vi "KickToSkill.vi"(0 "KickToSkill in":refnum<class "KickToSkill.lvclass">, 1 "use criteria?":bool, 2 "chipKick ?":bool, 5 "Robot":refnum<class "Robot.lvclass">, 9 "Game":refnum<class "Game.lvclass">, 10 "calculate force?":bool, 11 "error in (no error)":errorcluster, 12 "Target":dbl[](array[numeric]), 13 "KickForce 0?":bool) -> (4 "KickToSkill out":refnum<class "KickToSkill.lvclass">, 6 "Robot out":refnum<class "Robot.lvclass">, 15 "error out":errorcluster)   [LabVIEW 2020, in "KickToSkill.lvclass"]
uses:
  KickToSkill.lvclass
  Robot_class/Robot.lvclass
  Game_class/Game.lvclass
  Robot_class/roles.ctl
  Team_class/OffensivePlay.ctl
  Utilities_class/Utilities.lvclass
  Object_class/Object.lvclass/Object.ctl
  Robot_class/Robot.lvclass/Robot.ctl
  Game_class/Game.lvclass/Game.ctl
  Ball_class/Ball.lvclass/Ball.ctl
  Parameters_class/Parameters.lvclass/Parameters.ctl
  Team_class/Team.lvclass/Team.ctl
  <vilib>/Analysis/_algsub.llb/Real Vector Norm.vi
  <vilib>/Analysis/baseanly.llb/Real Dot Product.vi
  <vilib>/Analysis/coordinate.llb/2D Cartesian Coordinate Rotation (Scalar).vi
  Parameters_class/Read ChipKick Force 1.vi
  Team_class/Read OffensivePlay.vi
  Object_class/Read x.vi
  Robot_class/Write dest_x.vi
  Robot_class/Write dest_y.vi
  Robot_class/Write dest_orientation.vi
  Robot_class/Write kick_x.vi
  Robot_class/Write dest_x_kick.vi
  Robot_class/Write dest_y_kick.vi
  Robot_class/Write kick_z.vi
  Robot_class/Write dribble.vi
  Game_class/Read BallRef.vi
  Game_class/Read Parameters.lvclass.vi
  Game_class/Read FieldRef.vi
  Game_class/Read OffensiveTeam.vi
  Game_class/Read Utilities.lvclass.vi
  Game_class/Read EnemyRef.vi
  Parameters_class/Read ShootOutForce.vi
  Parameters_class/Read AttakingOurselves.vi
  Parameters_class/Read KickEps.vi
  Parameters_class/Read KickRange.vi
  Parameters_class/Read MinDistToKick.vi
  Parameters_class/Read DistanceToKickingAngle.vi
  Parameters_class/Read Force++.vi
  Parameters_class/Read ChipKick activated.vi
  Parameters_class/Read KickAngle.vi
  Parameters_class/Read DistanceToGoAroundBall.vi
  Parameters_class/Read KickForce.vi
  Parameters_class/Read Shoot Out_.vi
  Object_class/Read y.vi
  Ball_class/Read v_x.vi
  Ball_class/Read v_y.vi
  Robot_class/Read role.vi
  Robot_class/Read orientation.vi
  Ally_class/Ally.lvclass
  Ball_class/Ball.lvclass
  Parameters_class/Parameters.lvclass
  Field_class/Field.lvclass
  Enemy_class/Enemy.lvclass
  <vilib>/Analysis/NI_AALPro.lvlib
  <vilib>/Analysis/NI_AALBase.lvlib
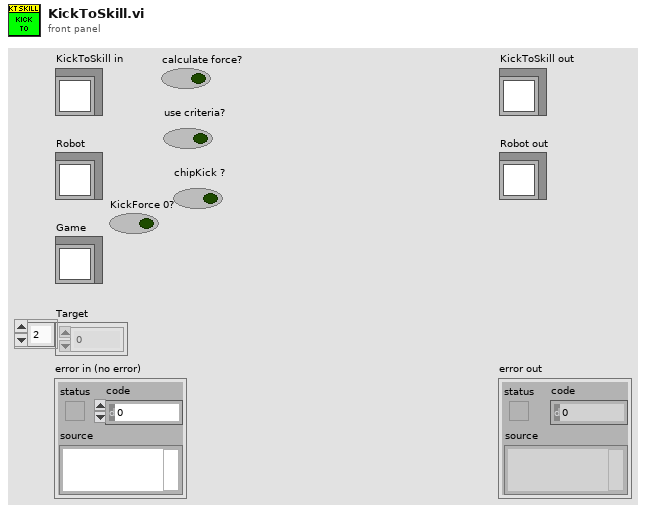
[diagram p1: front panel]
types:
  T1 = typedef "OffensivePlay.ctl" = enum16{"ABCPass", "PrepareTriplePass", "TableWithStriker", "TableWith2ndStrikerPlay", "PrepareDoublePass", "PrepareRollToPass", "SimplePass", "PreparePass", "PassToStriker", "BallOutOfField", "PassTo2ndStriker", "StopOffensive", "Prepare Penalty Enemy", "EnemyPossessionAtEnemyField", "EnemyPossesionAtOurField", "TestPlay", "PreparePenaltyAlly", "KickPenaltyAlly", "PrepareKickoffAlly", "PrepareKickoffEnemy", "IndirectEnemy", "DirectEnemy", "PreparePassInGame1", "NormalGame", "DirectKick", "Pass", "Halt", "Timeout", "PassPlay", "PenaltyEnemy"}
  T2 = typedef "roles.ctl" = enum16{"ABCThirdKicker", "ABCFirstKicker", "ABCSecondKicker", "Tabler", "TableFinalizer", "PrepareRollToPassRoller", "PrepareRollToPassReceiver", "SimplePassRoll", "SimplePassRollReceiver", "PenaltyDefense", "PreparePassReceiver 2", "PreparePassReceiver 1", "PassObserver", "Timeout", "Goto", "ZigZag", "None", "BallOutOfField", "DefenderArea", "Duelist", "AttackerStop", "FollowAttacker", "KeeperRole", "KickPenalty", "AttackerAimGoal", "AttackerBlock", "Marker", "Halt", "Shoot", "PassKicker", "PassReceiver", "TestRole", "PenaltyAttacker"}
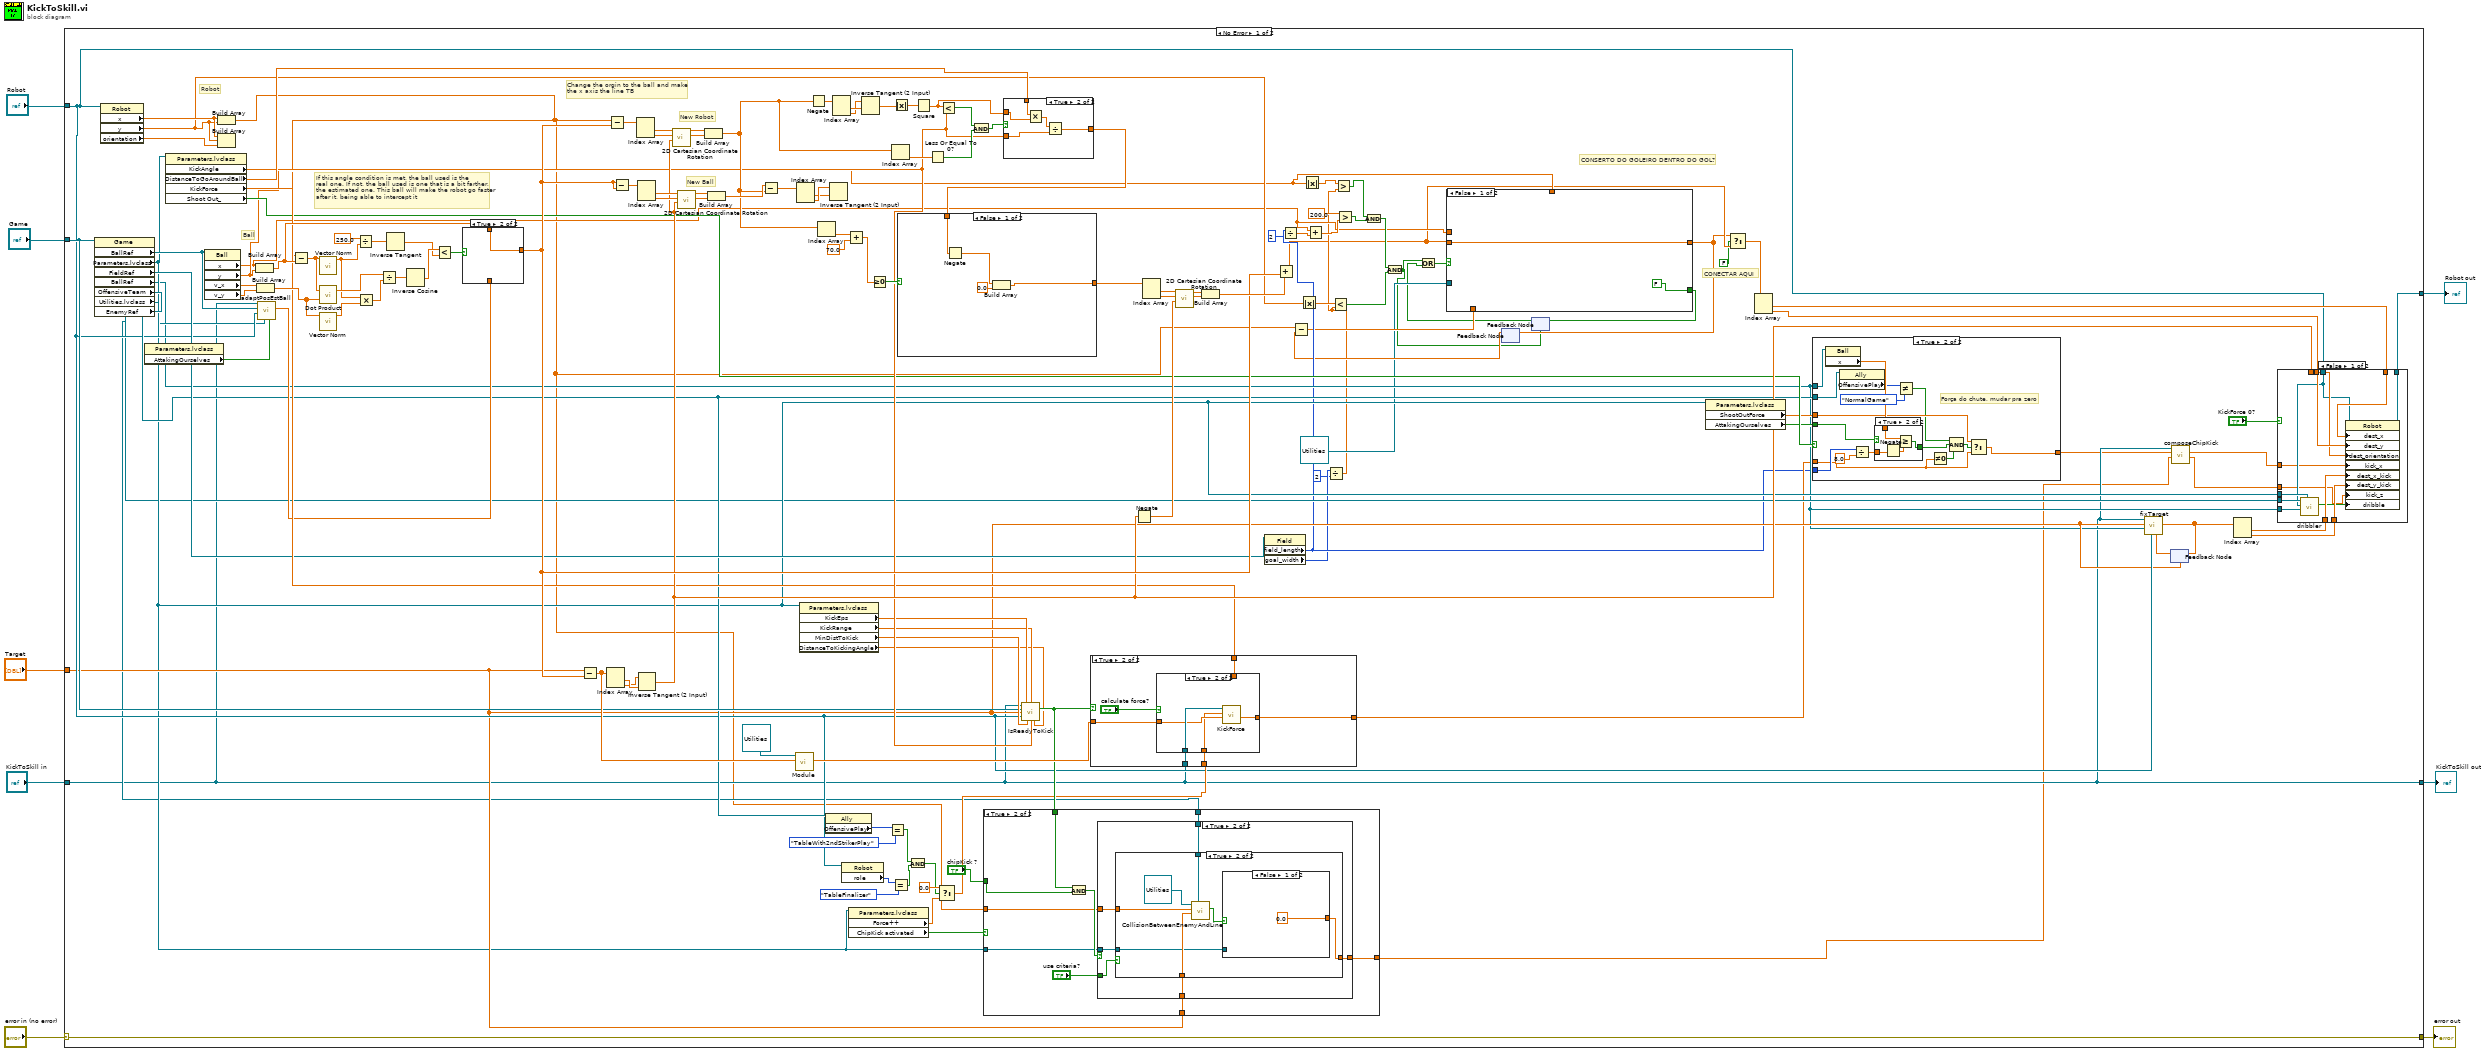
[diagram p0: block diagram]
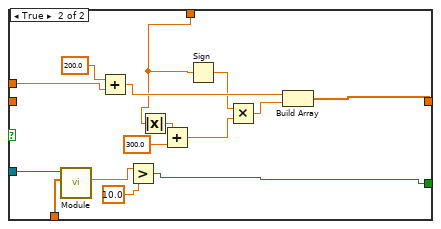
[diagram p2: hidden frame]
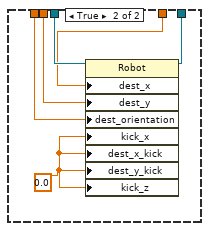
[diagram p3: hidden frame]
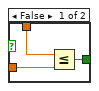
[diagram p5: hidden frame]
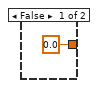
[diagram p6: hidden frame]
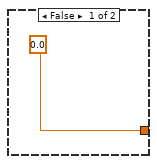
[diagram p7: hidden frame]
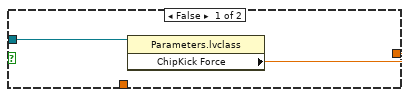
[diagram p8: hidden frame]
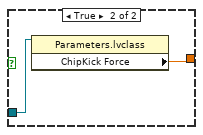
[diagram p9: hidden frame]
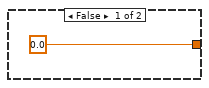
[diagram p10: hidden frame]
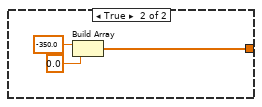
[diagram p12: hidden frame]
diagram:
  n1 = case shown="No Error" "error in (no error)" {
    selector: "error in (no error)" -> [w148 w267]
    tunnel: [w148 w267] -> w7
    tunnel: [w42 w266] -> w5
    tunnel: "KickToSkill in" -> [w42 w266]
    tunnel: "Robot" -> [w52 w265]
    tunnel: "Game" -> [w70 _]
    tunnel: "Target" -> [w49 _]
    tunnel: [w89 w265] -> w1
    frame No Error {
      # "CONECTAR AQUI"
      # "CONSERTO DO GOLEIRO DENTRO DO GOL?"
      # "Change the orgin to the ball and make \nthe x axis the line TB"
      # "If this angle condition is met, the ball used is the\nreal one. If not, the ball used is one that is a bit farther,\nthe estimated one. This ball will make the robot go faster\nafter it, being able to intercept it"
      # "New Robot"
      # "New Ball"
      # "Ball"
      # "Robot"
      n2 = property class="Game"(reference=w70) -> ("BallRef"=w68:refnum<class "Ball.lvclass">, "Parameters.lvclass"=w47:refnum<class "Parameters.lvclass">, "FieldRef"=w72:refnum<class "Field.lvclass">, "BallRef"=w45:refnum<class "Ball.lvclass">, "OffensiveTeam"=w57:refnum<class "Ally.lvclass">, "Utilities.lvclass"=w46:refnum<class "Utilities.lvclass">, "EnemyRef"=w43:refnum<class "Enemy.lvclass">)  [unwired: 1 in, 2 out]
      n3 = property class="Robot"(reference=w52) -> ("x"=w147:dbl, "y"=w34:dbl, "orientation"=w146:dbl)  [unwired: 1 in, 2 out]
      n4 = property class="Parameters.lvclass"(reference=w47) -> ("AttakingOurselves"=w66:bool)  [unwired: 1 in, 2 out]
      n5 = property class="Parameters.lvclass"(reference=w47) -> ("KickAngle"=w82:dbl, "DistanceToGoAroundBall"=w83:dbl, "KickForce"=w81:dbl, "Shoot Out_"=w71:bool)  [unwired: 1 in, 2 out]
      n6 = property class="Ball"(reference=w68) -> ("x"=w26:dbl, "y"=w30:dbl, "v_x"=w74:dbl, "v_y"=w73:dbl)  [unwired: 1 in, 2 out]
      n7 = Build Array(w147, w34) -> (w24:dbl[])
      n8 = Build Array(w147, w34, w146) -> ()  [unwired: 1 out]
      n9 = Build Array(w26, w30) -> (w95:dbl[])
      n10 = Build Array(w74, w73) -> (w144:dbl[])
      n11 = call "adaptPosEstBall.vi"("AttakingOurselves"=w66, "Utilities.lvclass"=w46, "Robot"=w52, "BallRef"=w68, "KickToSkill in"=w42) -> ("Pos_est adapted"=w69:dbl[])  [unwired: 4 in, 2 out]
      n12 = Subtract(x=w24, y=w95) -> (x-y=w145:dbl[])
      n13 = call-poly <vilib>:"Vector Norm.vi"("Input Vector"=w145) -> ("norm"=w139:dbl)  [unwired: 9 in, 1 out]
      n14 = call-poly <vilib>:"Dot Product.vi"("Y Vector"=w144, "X Vector"=w145) -> ("X * Y"=w142:dbl)  [unwired: 1 out]
      n15 = call-poly <vilib>:"Vector Norm.vi"("Input Vector"=w144) -> ("norm"=w143:dbl)  [unwired: 9 in, 1 out]
      n16 = Divide(x=250.0, y=w139) -> (x/y=w138:dbl)
      n17 = Multiply(x=w139, y=w143) -> (x*y=w141:dbl)
      n18 = Divide(x=w142, y=w141) -> (x/y=w137:dbl)
      n19 = Inverse Tangent(1:w138) -> (0:w135:dbl)
      n20 = Inverse Cosine(1:w137) -> (0:w136:dbl)
      n21 = Less?(x=w136, y=w135) -> (x < y?=w134:bool)
      n22 = case shown="True" w134 {
        tunnel: [w263 w264] -> w93
        tunnel: w95 -> [_ w264]
        tunnel: w69 -> [w263 _]
        frame False {
        }
        frame True {
        }
      }
      n23 = Subtract(x=w49, y=w93) -> (x-y=w88:dbl[])
      n24 = Index Array(array=w88) -> (element #1=w133:dbl, element #2=w132:dbl)  [unwired: 2 in]
      n25 = Subtract(x=w24, y=w93) -> (x-y=w131:dbl[])
      n26 = Subtract(x=w93, y=w93) -> (x-y=w128:dbl[])
      n27 = Index Array(array=w131) -> (element #1=w130:dbl, element #2=w129:dbl)  [unwired: 2 in]
      n28 = Index Array(array=w128) -> (element #1=w127:dbl, element #2=w126:dbl)  [unwired: 2 in]
      n29 = Inverse Tangent (2 Input)(1:w133, 2:w132) -> (0:w90:dbl)
      n30 = call-poly <vilib>:"2D Cartesian Coordinate Rotation.vi"("theta"=w90, "y"=w129, "x"=w130) -> ("y out"=w124:dbl, "x out"=w125:dbl)  [unwired: 6 in, 1 out]
      n31 = call-poly <vilib>:"2D Cartesian Coordinate Rotation.vi"("theta"=w90, "y"=w126, "x"=w127) -> ("y out"=w122:dbl, "x out"=w123:dbl)  [unwired: 6 in, 1 out]
      n32 = Build Array(w125, w124) -> (w110:dbl[])
      n33 = Build Array(w123, w122) -> (w121:dbl[])
      n34 = Subtract(x=w121, y=w110) -> (x-y=w118:dbl[])
      n35 = call-dynamic "Module.vi"("2D vector"=w88, "Utilities in"=refnum<class "Utilities.lvclass"> refnum) -> ("Modulo"=w86:dbl)  [unwired: 7 in, 2 out]
      n36 = Index Array(array=w118) -> (element #1=w119:dbl, element #2=w120:dbl)  [unwired: 2 in]
      n37 = property class="Parameters.lvclass"(reference=w47) -> ("KickEps"=w78:dbl, "KickRange"=w77:dbl, "MinDistToKick"=w76:dbl, "DistanceToKickingAngle"=w75:dbl)  [unwired: 1 in, 2 out]
      n38 = Negate(x=w110) -> (-x=w115:dbl[])
      n39 = Index Array(array=w110) -> (element=w117:dbl)  [unwired: 1 in]
      n40 = property class="Ally"(reference=w57) -> ("OffensivePlay"=w56:T1)  [unwired: 1 in, 2 out]
      n41 = Inverse Tangent (2 Input)(1:w119, 2:w120) -> ()  [unwired: 1 out]
      n42 = Index Array(array=w115) -> (element #1=w114:dbl, element #2=w113:dbl)  [unwired: 2 in]
      n43 = property class="Robot"(reference=w52) -> ("role"=w60:T2)  [unwired: 1 in, 2 out]
      n44 = Add(x=w117, y=70.0) -> (x+y=w104:dbl)
      n45 = property class="Parameters.lvclass"(reference=w47) -> ("Force++"=w63:dbl, "ChipKick activated"=w79:bool)  [unwired: 1 in, 2 out]
      n46 = Inverse Tangent (2 Input)(1:w114, 2:w113) -> (0:w112:dbl)
      n47 = Greater Or Equal To 0?(x=w104) -> (x >= 0?=w103:bool)
      n48 = Equal?(x=w56, y=OffensivePlay."TableWith2ndStrikerPlay") -> (x = y?=w54:bool)
      n49 = Index Array(array=w110) -> (element=w109:dbl)  [unwired: 1 in]
      n50 = Equal?(x=w60, y=roles."TableFinalizer") -> (x = y?=w58:bool)
      n51 = Absolute Value(x=w112) -> (abs(x)=w111:dbl)
      n52 = And(x=w54, y=w58) -> (x .and. y?=w53:bool)
      n53 = Square(x=w111) -> (x^2=w105:dbl)
      n54 = Less Or Equal To 0?(x=w109) -> (x <= 0?=w107:bool)
      n55 = Select(t=0.0, s=w53, f=w63) -> (s? t:f=w62:dbl)
      n56 = Less?(x=w105, y=w82) -> (x < y?=w108:bool)
      n57 = And(x=w108, y=w107) -> (x .and. y?=w106:bool)
      n58 = case shown="True" w106 {
        tunnel: w83 -> [w257 w262]
        tunnel: w105 -> [_ w261]
        tunnel: w82 -> [_ w259]
        tunnel: [w257 w258] -> w102
        frame False {
        }
        frame True {
          n59 = Multiply(x=w262, y=w261) -> (x*y=w260:dbl)
          n60 = Divide(x=w260, y=w259) -> (x/y=w258:dbl)
        }
      }
      n61 = case shown="False" w103 {
        tunnel: [w250 w254] -> w101
        tunnel: w102 -> [w252 _]
        frame False {
          n62 = Negate(x=w252) -> (-x=w251:dbl)
          n63 = Build Array(w251, 0.0 ("element")) -> (w250:dbl[])
        }
        frame True {
          n64 = Build Array(-350.0 ("element"), 0.0 ("element")) -> (w254:dbl[])
        }
      }
      n65 = call-dynamic "IsReadyToKick.vi"("KickToSkill in"=w42, "KickEps"=w78, "KickRange"=w77, "Game"=w70, "Target"=w49, "Robot"=w52, "MinDistToKick"=w76, "KickingAngle"=w82, "DistToKickingAngle"=w75) -> ("CanKick?"=w80:bool)  [unwired: 4 in, 2 out]
      n66 = case shown="True" w79 {
        tunnel: [0.0 ("ChipKick Force") w218] -> w39
        tunnel: w80 -> [_ w216]
        tunnel: w24 -> [_ w214]
        tunnel: w49 -> [_ w213]
        tunnel: w47 -> [_ w212]
        tunnel: "chipKick ?" -> [_ w211]
        tunnel: w43 -> [_ w210]
        frame False {
        }
        frame True {
          n67 = And(x=w216, y=w211) -> (x .and. y?=w215:bool)
          n68 = case shown="True" w215 {
            tunnel: [0.0 w223] -> w218
            tunnel: "use criteria?" -> [_ w225]
            tunnel: w212 -> [_ w224]
            tunnel: w214 -> [_ w222]
            tunnel: w213 -> [_ w221]
            tunnel: w210 -> [_ w220]
            frame False {
            }
            frame True {
              n69 = case shown="True" w225 {
                tunnel: w224 -> [w227 w229]
                tunnel: [w226 w230] -> w223
                tunnel: w222 -> [_ w233]
                tunnel: w221 -> [_ w232]
                tunnel: w220 -> [_ w228]
                frame False {
                  n70 = property class="Parameters.lvclass"(reference=w227) -> ("ChipKick Force"=w226:dbl)  [unwired: 1 in, 2 out]
                }
                frame True {
                  n71 = call-dynamic "CollisionBetweenEnemyAndLine.vi"("EnemyRef"=w228, "P2"=w232, "P1"=w233, "Utilities in"=refnum<class "Utilities.lvclass"> refnum) -> ("collision ?"=w231:bool)  [unwired: 4 in, 3 out]
                  n72 = case shown="False" w231 {
                    tunnel: [0.0 w237] -> w230
                    tunnel: w229 -> [_ w236]
                    frame False {
                    }
                    frame True {
                      n73 = property class="Parameters.lvclass"(reference=w236) -> ("ChipKick Force"=w237:dbl)  [unwired: 1 in, 2 out]
                    }
                  }
                }
              }
            }
          }
        }
      }
      n74 = case shown="True" w80 {
        tunnel: w42 -> [_ w243]
        tunnel: [0.0 ("Force") w239] -> w44
        tunnel: w86 -> [_ w242]
        tunnel: w81 -> [_ w241]
        tunnel: w62 -> [_ w240]
        frame False {
        }
        frame True {
          n75 = case shown="True" "calculate force?" {
            tunnel: w243 -> [_ w249]
            tunnel: [w245 w248] -> w239
            tunnel: w242 -> [_ w247]
            tunnel: w241 -> [w245 _]
            tunnel: w240 -> [_ w246]
            frame False {
            }
            frame True {
              n76 = call-dynamic "KickForce.vi"("Distance to target"=w247, "force++"=w246, "KickToSkill in"=w249) -> ("Force"=w248:dbl)  [unwired: 6 in, 2 out]
            }
          }
        }
      }
      n77 = Negate(x=w90) -> (-x=w98:dbl)
      n78 = Index Array(array=w101) -> (element #1=w99:dbl, element #2=w100:dbl)  [unwired: 2 in]
      n79 = call-poly <vilib>:"2D Cartesian Coordinate Rotation.vi"("theta"=w98, "y"=w100, "x"=w99) -> ("y out"=w96:dbl, "x out"=w97:dbl)  [unwired: 6 in, 1 out]
      n80 = Build Array(w97, w96) -> (w94:dbl[])
      n81 = property class="Field"(reference=w72) -> ("field_length"=w37:i32, "goal_width"=w20:i32)  [unwired: 1 in, 2 out]
      n82 = Add(x=w94, y=w93) -> (x+y=w14:dbl[])
      n83 = Divide(x=w37, y=2) -> (x/y=w35:dbl)
      n84 = Absolute Value(x=w34) -> (abs(x)=w33:dbl)
      n85 = Absolute Value(x=w30) -> (abs(x)=w18:dbl)
      n86 = Add(x=w26, y=w35) -> (x+y=w27:dbl)
      n87 = Divide(x=w20, y=2) -> (x/y=w17:dbl)
      n88 = Less?(x=w33, y=w17) -> (x < y?=w32:bool)
      n89 = Greater?(x=w18, y=w17) -> (0:w16:bool)
      n90 = Greater?(x=200.0, y=w27) -> (0:w28:bool)
      n91 = And(x=w16, y=w28) -> (x .and. y?=w31:bool)
      n92 = And(x=w31, y=w32) -> (x .and. y?=w12:bool)
      n93 = feedback #1() -> (w25:dbl[])  [unwired: 1 in]
      n94 = Subtract(x=w24, y=w25) -> (x-y=w23:dbl[])
      n95 = feedback #2(w12) -> (w11:bool)
      n96 = Or(x=w12, y=w11) -> (x .or. y?=w10:bool)
      n97 = case shown="False" w10 {
        tunnel: w14 -> [w150 _]
        tunnel: [w150 w162] -> w13
        tunnel: w30 -> [_ w157]
        tunnel: w26 -> [_ w165]
        tunnel: w23 -> [_ w161]
        tunnel: refnum<class "Utilities.lvclass"> refnum ("Utilities in") -> [_ w160]
        tunnel: [FALSE w151] -> w15
        frame False {
        }
        frame True {
          n98 = call-dynamic "Module.vi"("2D vector"=w161, "Utilities in"=w160) -> ("Modulo"=w153:dbl)  [unwired: 7 in, 2 out]
          n99 = Add(x=200.0, y=w165) -> (x+y=w163:dbl)
          n100 = Greater?(x=w153, y=10.0) -> (0:w151:bool)
          n101 = Absolute Value(x=w157) -> (abs(x)=w159:dbl)
          n102 = Add(x=w159, y=300.0) -> (x+y=w156:dbl)
          n103 = Sign(1:w157) -> (0:w155:dbl)
          n104 = Multiply(x=w155, y=w156) -> (x*y=w154:dbl)
          n105 = Build Array(w163, w154) -> (w162:dbl[])
        }
      }
      n106 = feedback-in #1(w13) -> ()
      n107 = feedback-in #2(w15) -> ()
      n108 = property class="Parameters.lvclass"(reference=w47) -> ("ShootOutForce"=w65:dbl, "AttakingOurselves"=w64:bool)  [unwired: 1 in, 2 out]
      n109 = Select(t=w13, s=FALSE, f=w14) -> (s? t:f=w21:dbl[])
      n110 = Index Array(array=w21) -> (element #1=w92:dbl, element #2=w91:dbl)  [unwired: 2 in]
      n111 = case shown="True" w71 {
        tunnel: w37 -> [_ w201]
        tunnel: w45 -> [_ w198]
        tunnel: w44 -> [w185 w193]
        tunnel: [w185 w196] -> w41
        tunnel: w65 -> [_ w191]
        tunnel: w64 -> [_ w190]
        tunnel: w57 -> [_ w186]
        frame False {
        }
        frame True {
          # "Força do chute, mudar pra zero"
          n112 = property class="Ball"(reference=w198) -> ("x"=w197:dbl)  [unwired: 1 in, 2 out]
          n113 = property class="Ally"(reference=w186) -> ("OffensivePlay"=w189:T1)  [unwired: 1 in, 2 out]
          n114 = Divide(x=w201, y=8.0) -> (x/y=w199:dbl)
          n115 = case shown="True" w190 {
            tunnel: w199 -> [w204 w208]
            tunnel: w197 -> [w203 w205]
            tunnel: [w202 w207] -> w194
            frame False {
              n116 = Less Or Equal?(x=w203, y=w204) -> (x <= y?=w202:bool)
            }
            frame True {
              n117 = Negate(x=w208) -> (-x=w206:dbl)
              n118 = Greater Or Equal?(x=w205, y=w206) -> (x >= y?=w207:bool)
            }
          }
          n119 = Not Equal?(x=w189, y=OffensivePlay."NormalGame") -> (x != y?=w187:bool)
          n120 = Not Equal To 0?(x=w193) -> (x != 0?=w192:bool)
          n121 = Compound Arithmetic op=AND(w187, w194, w192) -> (w195:bool)
          n122 = Select(t=w191, s=w195, f=w193) -> (s? t:f=w196:dbl)
        }
      }
      n123 = feedback #3(w49) -> (w50:dbl[])
      n124 = call "fixTarget.vi"("LastTarget"=w50, "Robot"=w52, "Ball"=w45, "Target in"=w49, "KickToSkill in"=w42) -> ("Target out"=w51:dbl[])  [unwired: 4 in, 2 out]
      n125 = feedback-in #3(w51) -> ()
      n126 = call "composeChipKick.vi"("kick_z"=w39, "kick_x"=w41, "KickToSkill in"=w42) -> ("kick_z out"=w38:dbl, "kick_x out"=w40:dbl)  [unwired: 5 in, 2 out]
      n127 = Index Array(array=w51) -> (element #1=w85:dbl, element #2=w84:dbl)  [unwired: 2 in]
      n128 = case shown="False" "KickForce 0?" {
        tunnel: w92 -> [w178 w182]
        tunnel: w91 -> [w177 w180]
        tunnel: w90 -> [w176 w179]
        tunnel: [w175 w184] -> w89
        tunnel: w52 -> [w169 w183]
        tunnel: w85 -> [w174 _]
        tunnel: w84 -> [w173 _]
        tunnel: w47 -> [w171 _]
        tunnel: w46 -> [w170 _]
        tunnel: w45 -> [w168 _]
        tunnel: w40 -> [w167 _]
        tunnel: w38 -> [w166 _]
        frame False {
          n129 = call "dribbler.vi"("Parameters.lvclass"=w171, "Ball"=w168, "Robot"=w169, "Utilities in"=w170) -> ("Dribbler?"=w172:bool)  [unwired: 5 in, 2 out]
          n130 = property class="Robot"(reference=w169, "dest_x"=w178, "dest_y"=w177, "dest_orientation"=w176, "kick_x"=w167, "dest_x_kick"=w174, "dest_y_kick"=w173, "kick_z"=w166, "dribble"=w172) -> (reference out=w175:refnum<class "Robot.lvclass">)  [unwired: 1 in, 1 out]
        }
        frame True {
          w181 = 0.0 ("Best y")
          n131 = property class="Robot"(reference=w183, "dest_x"=w182, "dest_y"=w180, "dest_orientation"=w179, "kick_x"=w181, "dest_x_kick"=w181, "dest_y_kick"=w181, "kick_z"=w181) -> (reference out=w184:refnum<class "Robot.lvclass">)  [unwired: 1 in, 1 out]
        }
      }
    }
    frame Error {
    }
  }
  "error out" <- w7
  "KickToSkill out" <- w5
  "Robot out" <- w1
